vi "apply channel changes.vi"(8 "error in":errorcluster, 9 "new":refnum<class "EIP Tags Channel.lvclass">, 10 "old":refnum<class "EIP Tags Channel.lvclass">, 11 "EthernetIP configuration in":refnum<class "EIP Tags Configuration.lvclass">) -> (0 "error out":errorcluster, 3 "EthernetIP configuration out":refnum<class "EIP Tags Configuration.lvclass">)   [LabVIEW 2013, in "EIP Tags Configuration.lvclass"]
uses:
  EIP Tags Configuration.lvclass
  channel/EIP Tags Channel.lvclass
  <vilib>/NI/Tag Bus/tag/tag descriptor.lvclass
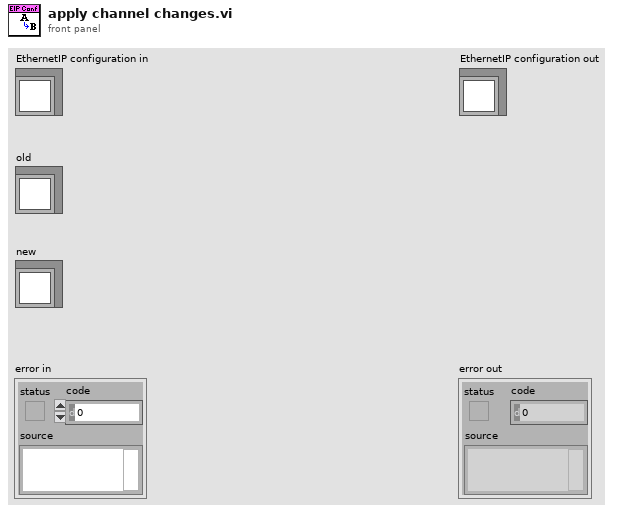
[diagram p1: front panel]
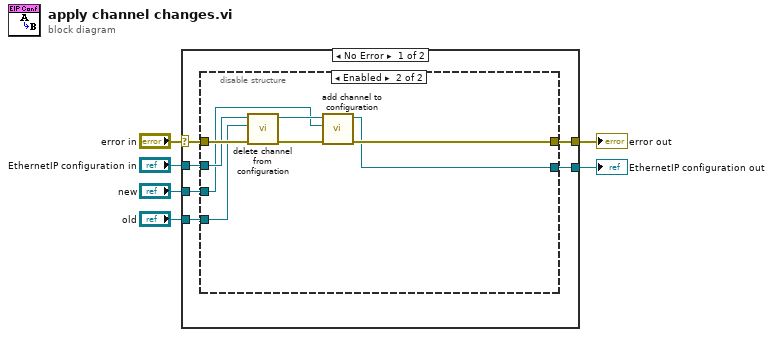
[diagram p0: block diagram]
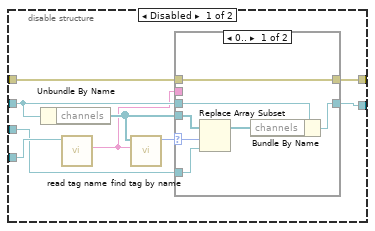
[diagram p2: hidden frame]
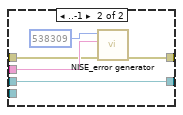
[diagram p3: hidden frame]
diagram:
  n1 = case shown="No Error" "error in" {
    selector: "error in" -> [w8 w43]
    tunnel: [w7 w43] -> w5
    tunnel: [w10 w42] -> w3
    tunnel: "EthernetIP configuration in" -> [w11 w42]
    tunnel: "old" -> [w12 _]
    tunnel: "new" -> [w9 _]
    frame No Error {
      n2 = disable-structure shown="Enabled" {
        disable-tunnel: w12 -> [w21 w35]
        disable-tunnel: w11 -> [w20 w37]
        disable-tunnel: [w19 w36] -> w10
        disable-tunnel: w9 -> [w17 w34]
        disable-tunnel: w8 -> [w16 w40]
        disable-tunnel: [w15 w39] -> w7
        frame Disabled {
          n3 = Unbundle By Name(w20) -> ("channels"=w18:refnum<class "EIP Tags Channel.lvclass">[])
          n4 = call <vilib>:"read tag name.vi"("system tag in"=w21) -> ("name"=w13:string)  [unwired: 8 in, 2 out]
          n5 = call <vilib>:"find tag by name.vi"("name"=w13, "tags in"=w18) -> ("index"=w14:i32)  [unwired: 9 in]
          n6 = case shown="0.." w14 {
            selector: w14 -> [w26 _]
            tunnel: w20 -> [w28 w33]
            tunnel: [w25 w33] -> w19
            tunnel: w18 -> [w27 _]
            tunnel: w17 -> [w23 _]
            tunnel: w13 -> [_ w31]
            tunnel: w16 -> [w22 w30]
            tunnel: [w22 w29] -> w15
            frame 0.. {
              n7 = Replace Array Subset(array=w27, new element=w23, index=w26) -> (w24:refnum<class "EIP Tags Channel.lvclass">[])
              n8 = Bundle By Name(cluster=w28, "channels"=w24) -> (w25:refnum<class "EIP Tags Configuration.lvclass">)
            }
            frame ..-1 {
              n9 = call <vilib>:"NISE_error generator.vi"("error in"=w30, "append error message"=w31, "error code (0)"=538309) -> ("error out"=w29:errorcluster)  [unwired: 6 in]
            }
          }
        }
        frame Enabled {
          n10 = call "delete channel from configuration.vi"("error in"=w40, "TBM channel in"=w35, "EthernetIP configuration in"=w37) -> ("error out"=w41:errorcluster, "EthernetIP configuration out"=w38:refnum<class "EIP Tags Configuration.lvclass">)  [unwired: 7 in]
          n11 = call "add channel to configuration.vi"("error in"=w41, "TBM channel in"=w34, "EthernetIP configuration in"=w38) -> ("error out"=w39:errorcluster, "EthernetIP configuration out"=w36:refnum<class "EIP Tags Configuration.lvclass">)  [unwired: 7 in]
        }
      }
    }
    frame Error {
    }
  }
  "error out" <- w5
  "EthernetIP configuration out" <- w3
